vi "JSON BAT.vi"(7 "Numeric":dbl, 8 "error in":errorcluster, 9 "Numeric 2":dbl, 10 "Numeric 3":dbl, 11 "JSON Object in":refnum<class "JSON Object.lvclass">) -> (0 "error out":errorcluster, 3 "JSON Object out":refnum<class "JSON Object.lvclass">)   [LabVIEW 2015]
uses:
  <vilib>/addons/JSON API/Get Polymorphic/JSON GetSet.lvlib
  <vilib>/addons/JSON API/JSON Scalar/Set SGL.vi
  <vilib>/addons/JSON API/JSON Scalar/JSON Scalar.lvclass
  <vilib>/addons/JSON API/JSON Object/Set Object Item by name.vi
  <vilib>/addons/JSON API/JSON Object/JSON Object.lvclass
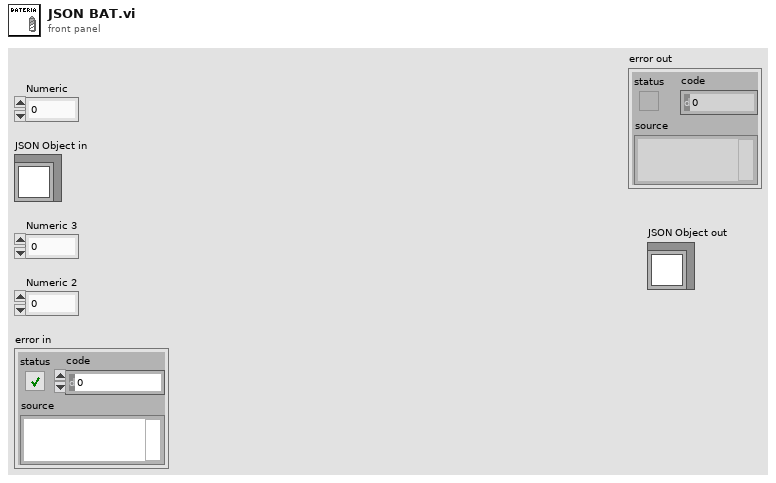
[diagram p1: front panel]
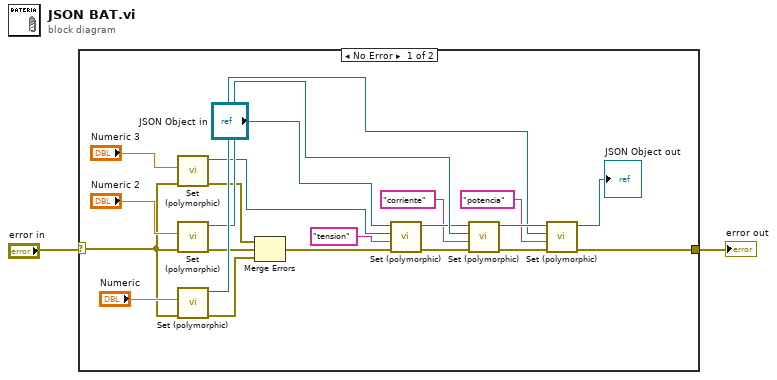
[diagram p0: block diagram]
diagram:
  n1 = case shown="No Error" "error in" {
    selector: "error in" -> [w3 w24]
    tunnel: [w5 w24] -> w2
    frame No Error {
      n2 = call-poly <vilib>:"Set (polymorphic).vi"("error in (no error)"=w3, "Numeric"="Numeric 3") -> ("error out"=w11:errorcluster, "JSON Scalar out"=w14:refnum<class "JSON Scalar.lvclass">)  [unwired: 8 in]
      n3 = call-poly <vilib>:"Set (polymorphic).vi"("error in (no error)"=w3, "Numeric"="Numeric 2") -> ("error out"=w10:errorcluster, "JSON Scalar out"=w19:refnum<class "JSON Scalar.lvclass">)  [unwired: 8 in]
      n4 = call-poly <vilib>:"Set (polymorphic).vi"("error in (no error)"=w3, "Numeric"="Numeric") -> ("error out"=w9:errorcluster, "JSON Scalar out"=w21:refnum<class "JSON Scalar.lvclass">)  [unwired: 8 in]
      n5 = Merge Errors(w11, w10, w9) -> (w8:errorcluster)
      n6 = call-poly <vilib>:"Set (polymorphic).vi"("error in (no error)"=w8, "name"="tension", "Value"=w14, "JSON Object in"="JSON Object in") -> ("error out"=w7:errorcluster, "JSON Object out"=w17:refnum<class "JSON Object.lvclass">)  [unwired: 5 in, 1 out]
      n7 = call-poly <vilib>:"Set (polymorphic).vi"("error in (no error)"=w7, "name"="corriente", "Value"=w19, "JSON Object in"=w17) -> ("error out"=w6:errorcluster, "JSON Object out"=w22:refnum<class "JSON Object.lvclass">)  [unwired: 5 in, 1 out]
      n8 = call-poly <vilib>:"Set (polymorphic).vi"("error in (no error)"=w6, "name"="potencia", "Value"=w21, "JSON Object in"=w22) -> ("error out"=w5:errorcluster, "JSON Object out"=→"JSON Object out":refnum<class "JSON Object.lvclass">)  [unwired: 5 in, 1 out]
    }
    frame Error {
    }
  }
  "error out" <- w2
